vi "DSF Transfer Group.Retrieve from FIFO.vi"(8 "error in (no error)":errorcluster, 9 "timeout in ms (0)":i32 format="%d ms", 10 "expected iteration":u64, 11 "Transfer Group in":refnum<class "Transfer Group.lvclass">) -> (0 "error out":errorcluster, 2 "iteration valid?":bool, 3 "Transfer Group out":refnum<class "Transfer Group.lvclass">)   [LabVIEW 2017, in "DSF Core.lvlib" / "Transfer Group.lvclass"]
uses:
  Transfer Group.lvclass
  Transfer Group.lvclass/Transfer Group.ctl
  Debug/Debug Flags/Debug Flags.lvclass/Debug Flags.ctl
  Debug/FIFO Flags/FIFO Flags.lvclass/FIFO Flags.ctl
  Transfer Group.Get Return FIFO.vi
  Transfer Group.Get Debug Flags.vi
  Debug/Debug Flags/Get FIFO Flags.vi
  Debug/FIFO Flags/Get Infinite Timeouts.vi
  Transfer Group.Errors.Return Timeout.vi
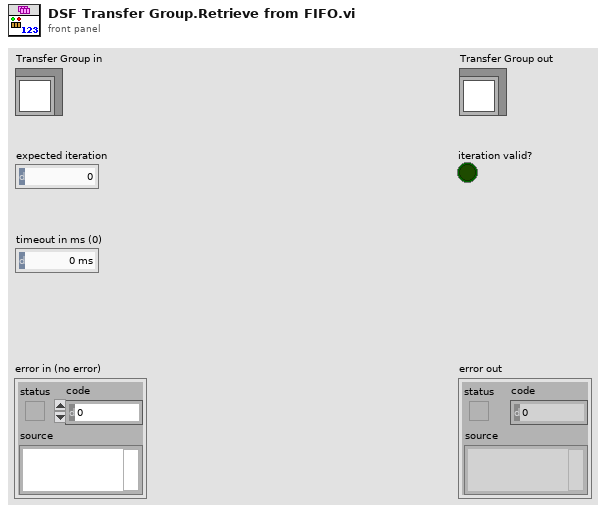
[diagram p1: front panel]
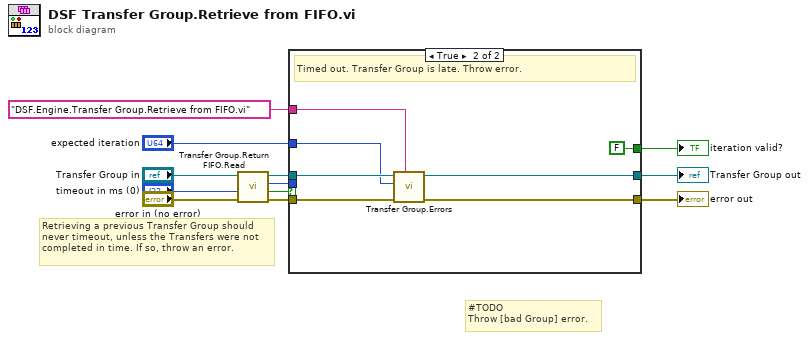
[diagram p0: block diagram]
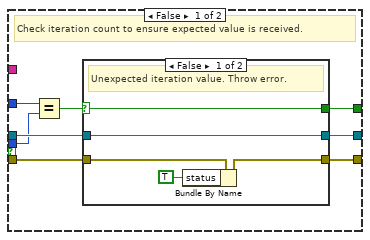
[diagram p2: hidden frame]
diagram:
  # "#TODO\nThrow [bad Group] error."
  # "Retrieving a previous Transfer Group should never timeout, unless the Transfers were not completed in time. If so, throw an error."
  n1 = call "Transfer Group.Return FIFO.Read.vi"("error in (no error)"="error in (no error)", "timeout in ms (0)"="timeout in ms (0)", "Transfer Group in"="Transfer Group in") -> ("error out"=w12:errorcluster, "timed out?"=w11:bool, "Transfer Group iteration"=w9:u64, "Transfer Group out"=w10:refnum<class "Transfer Group.lvclass">)  [unwired: 5 in]
  n2 = case shown="True" w11 {
    tunnel: w12 -> [w16 w33]
    tunnel: w10 -> [w18 w34]
    tunnel: w9 -> [w14 _]
    tunnel: "expected iteration" -> [w20 w32]
    tunnel: [w15 w29] -> w4
    tunnel: [w17 w30] -> w5
    tunnel: [w13 FALSE] -> w3
    tunnel: "DSF.Engine.Transfer Group.Retrieve from FIFO.vi" ("error source vi name") -> [_ w31]
    frame False {
      # "Check iteration count to ensure expected value is received."
      n3 = Equal?(x=w20, y=w14) -> (x = y?=w19:bool)
      n4 = case shown="False" w19 {
        selector: w19 -> [w21 w26]
        tunnel: w18 -> [w25 w28]
        tunnel: [w25 w28] -> w17
        tunnel: w16 -> [w24 w27]
        tunnel: [w23 w27] -> w15
        tunnel: [w21 w26] -> w13
        frame False {
          # "Unexpected iteration value. Throw error."
          n5 = Bundle By Name(cluster=w24, "status"=TRUE) -> (w23:errorcluster)
        }
        frame True {
          # "Expected value. Proceed."
        }
      }
    }
    frame True {
      # "Timed out. Transfer Group is late. Throw error."
      n6 = call-poly "Transfer Group.Errors.vi"("error source vi name"=w31, "error in (no error)"=w33, "expected iteration"=w32, "Transfer Group in"=w34) -> ("error out"=w29:errorcluster, "Transfer Group out"=w30:refnum<class "Transfer Group.lvclass">)  [unwired: 6 in]
    }
  }
  "error out" <- w4
  "Transfer Group out" <- w5
  "iteration valid?" <- w3
